vi "FTW-JSON-ObjectManip-AddPair-Element.vi"(0 "Input JSON Object":string, 5 "Key":string, 7 "Element String":string, 11 "error in":errorcluster) -> (4 "Output JSON Object":string, 15 "error out":errorcluster)   [LabVIEW 2013]
panel:
  # "Inputs"
  # "Outputs"
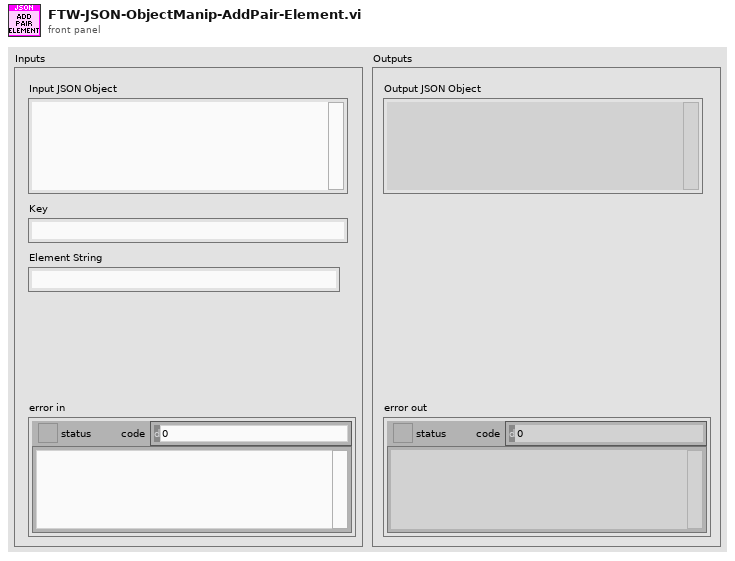
[diagram p1: front panel]
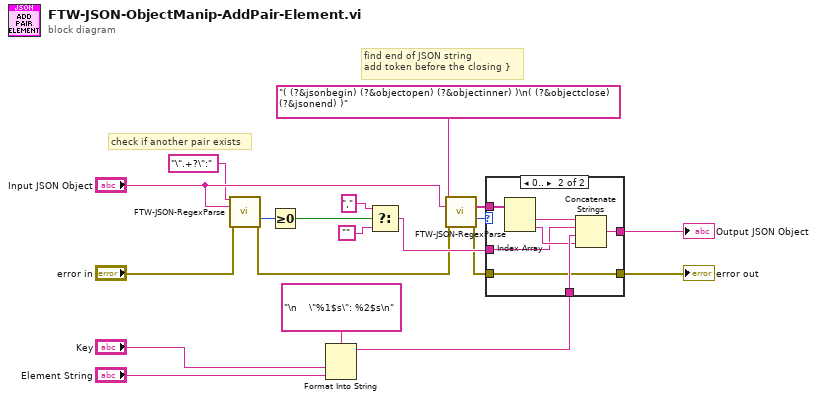
[diagram p0: block diagram]
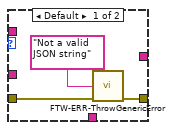
[diagram p2: hidden frame]
diagram:
  # "find end of JSON string\nadd token before the closing }"
  # "check if another pair exists"
  n1 = call "FTW-JSON-RegexParse.vi"("Regular Expression using JSON subroutines"="\".+?\":" ("format string"), "Input String"="Input JSON Object", "error in"="error in") -> ("Offset after Match"=w1:i32, "error out"=w6:errorcluster)  [unwired: 8 in, 3 out]
  n2 = Greater Or Equal To 0?(x=w1) -> (x >= 0?=w9:bool)
  n3 = Format Into String(format string="\n    \"%1$s\": %2$s\n", "Key", "Element String") -> (resulting string=w12:string)  [unwired: 2 in, 1 out]
  n4 = Select(t="," ("format string"), s=w9, f="") -> (s? t:f=w13:string)
  n5 = call "FTW-JSON-RegexParse.vi"("Regular Expression using JSON subroutines"="( (?&jsonbegin) (?&objectopen) (?&objectinner) )\n( (?&objectclose) (?&jsonend) )" ("format string"), "Input String"="Input JSON Object", "error in"=w6) -> ("Submatches"=w3:string[], "Offset after Match"=w2:i32, "error out"=w5:errorcluster)  [unwired: 8 in, 2 out]
  n6 = case shown="0.." w2 {
    tunnel: w3 -> [_ w29]
    tunnel: w12 -> [_ w27]
    tunnel: [_ w25] -> w14
    tunnel: w5 -> [w22 w24]
    tunnel: w13 -> [_ w23]
    tunnel: [w21 w24] -> w15
    frame Default {
      n7 = call "FTW-ERR-ThrowGenericError.vi"("Error Message"="Not a valid JSON string", "error in"=w22) -> ("error out"=w21:errorcluster)  [unwired: 13 in]
    }
    frame 0.. {
      n8 = Index Array(array=w29) -> (element #1=w28:string, element #2=w26:string)  [unwired: 2 in]
      n9 = Concatenate Strings(w28, w23, w27, w26) -> (w25:string)
    }
  }
  "error out" <- w15
  "Output JSON Object" <- w14
